vi "GV_YscaleLocatePlace.vi"(8 "error in (no error)":errorcluster, 9 "Pos":cluster{"x":i16, "y":i16}, 11 "Gviewer in":refnum<class "Gviewer.lvclass">) -> (0 "error out":errorcluster, 1 "Plot Images:Front":picture, 3 "Gviewer out":refnum<class "Gviewer.lvclass">)   [LabVIEW 2020, in "Sgraph_lib_V1.lvlib" / "Gviewer.lvclass"]
doc: "Andre Koelewijn, 27 April 2021\n\nMove legend over the graph area"
uses:
  Gviewer.lvclass
  <vilib>/Utility/miscctls.llb/LVPoint32TypeDef.ctl
  Gviewer.lvclass/Gviewer.ctl
panel:
  in  "Coords":T1
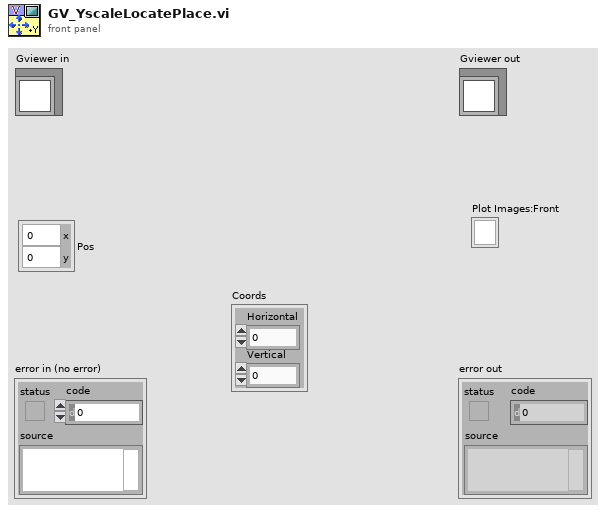
[diagram p1: front panel]
types:
  T1 = typedef "LVPoint32TypeDef.ctl" = cluster{"Horizontal":i32, "Vertical":i32}
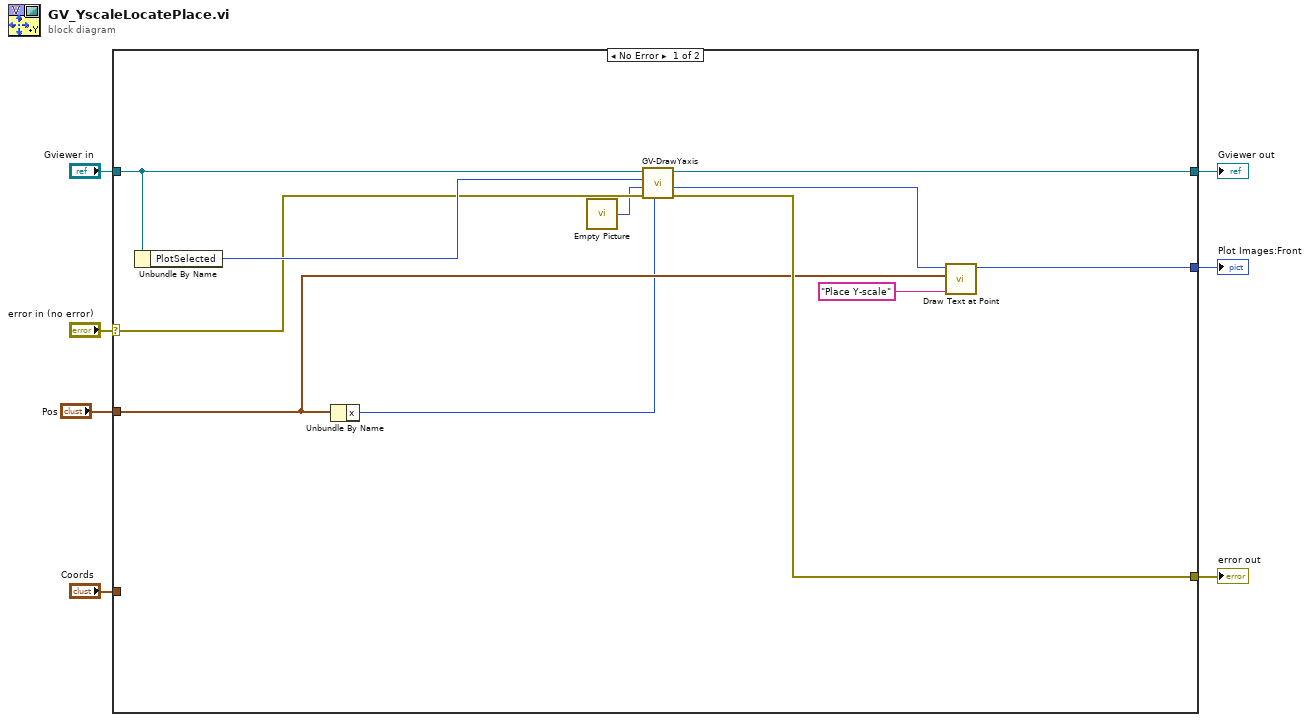
[diagram p0: block diagram]
diagram:
  n1 = case shown="No Error" "error in (no error)" {
    selector: "error in (no error)" -> [w16 w20]
    tunnel: [w17 w20] -> w6
    tunnel: [w14 w19] -> w4
    tunnel: "Gviewer in" -> [w15 w19]
    tunnel: "Coords" -> [_ _]
    tunnel: [w12 _] -> w2
    tunnel: "Pos" -> [w11 _]
    frame No Error {
      n2 = Unbundle By Name(w15) -> ("PlotSelected"=w18:i32)
      n3 = Unbundle By Name(w11) -> ("x"=w10:i16)
      n4 = call "Empty Picture"() -> ("empty picture"=w9:picture)
      n5 = call "GV-DrawYaxis.vi"("X-position"=w10, "error in (no error)"=w16, "Picture IN"=w9, "Plot"=w18, "Gviewer in"=w15) -> ("error out"=w17:errorcluster, "Picture OUT"=w8:picture, "Gviewer out"=w14:refnum<class "Gviewer.lvclass">)  [unwired: 4 in]
      n6 = call <vilib>:"Draw Text at Point.vi"("text"="Place Y-scale", "origin"=w11, "picture"=w8) -> ("new picture"=w12:picture)  [unwired: 7 in, 1 out]
    }
    frame Error {
    }
  }
  "error out" <- w6
  "Gviewer out" <- w4
  "Plot Images:Front" <- w2
